vi "RW_test_fullcycle.vi"() -> ()   [LabVIEW 2018]
panel:
  in  "voltage 2":dbl
  out "error out":errorcluster caption="Error OUT"
  in  "milliseconds to wait":u32=500
  in  "Rotating Wall Parameters":T1={"Start Frequency"=25000.0, "Stop Frequency"=26000.0, "Sweep Time"=10.0, "Amplitude"=0.0, "Phase (ch.1)"=0.0, "Phase (Ch.2)"=90.0} {"Sweep Time" format="%.4f"; "Phase (Ch.2)" min=-1800.0 max=1800.0 step=0.1 format="%.3f"; "Phase (ch.1)" min=-1800.0 max=1800.0 step=0.1 format="%.3f"; "Stop Frequency" format="%#.5p"; "Start Frequency" format="%#.5p"; "Amplitude" min=0.0 max=4.0 format="%.3f"}
  in  "voltage":dbl=2.0
  in  "VISAsession":refnum<visa-resource-name>="wavefactoryU5"
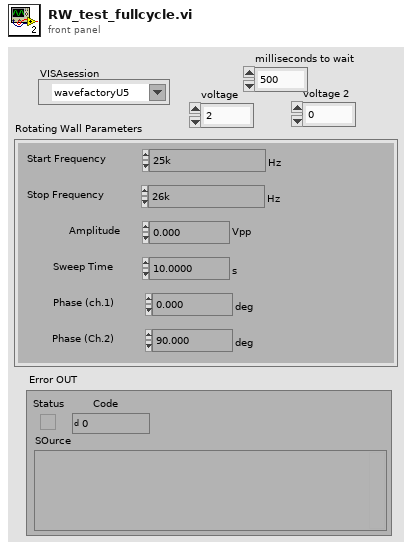
[diagram p1: front panel]
types:
  T1 = cluster{"Start Frequency":dbl, "Stop Frequency":dbl, "Sweep Time":dbl, "Amplitude":dbl, "Phase (ch.1)":dbl, "Phase (Ch.2)":dbl}
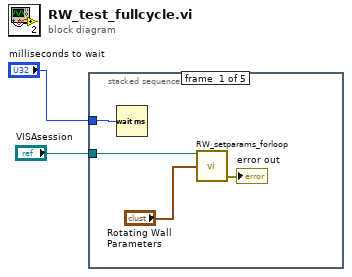
[diagram p0: block diagram]
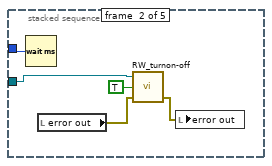
[diagram p2: hidden frame]
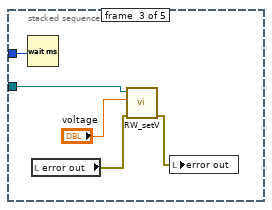
[diagram p3: hidden frame]
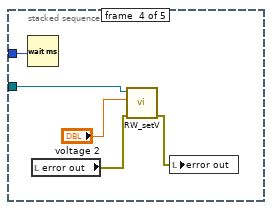
[diagram p4: hidden frame]
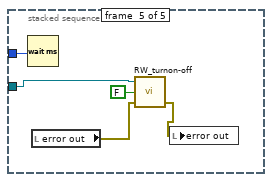
[diagram p5: hidden frame]
diagram:
  n1 = stacked-sequence {
    tunnel: "VISAsession" -> [w6 w10 w16 w21 w25]
    tunnel: "milliseconds to wait" -> [w4 w9 w15 w20 w24]
    frame #0 {
      n2 = Wait (ms)(milliseconds to wait=w4) -> ()  [unwired: 1 out]
      n3 = call "RW_setparams_forloop.vi"("Rotating Wall Parameters"="Rotating Wall Parameters", "VISAsession"=w6) -> ("error out"=→"error out":errorcluster)  [unwired: 2 in, 1 out]
    }
    frame #1 {
      n4 = Wait (ms)(milliseconds to wait=w9) -> ()  [unwired: 1 out]
      n5 = local read "error out"() -> (w8:errorcluster)
      n6 = call "RW_turnon-off.vi"("error in (no error)"=w8, "On/Off"=TRUE, "VISAsession"=w10) -> ("error out"=w7:errorcluster)  [unwired: 1 in, 1 out]
      n7 = local write "error out"(w7) -> ()
    }
    frame #2 {
      n8 = Wait (ms)(milliseconds to wait=w15) -> ()  [unwired: 1 out]
      n9 = local read "error out"() -> (w13:errorcluster)
      n10 = call "RW_setV.vi"("error in (no error)"=w13, "voltage"="voltage", "VISAsession"=w16) -> ("error out"=w12:errorcluster)  [unwired: 8 in]
      n11 = local write "error out"(w12) -> ()
    }
    frame #3 {
      n12 = Wait (ms)(milliseconds to wait=w20) -> ()  [unwired: 1 out]
      n13 = local read "error out"() -> (w18:errorcluster)
      n14 = call "RW_setV.vi"("error in (no error)"=w18, "voltage"="voltage 2", "VISAsession"=w21) -> ("error out"=w17:errorcluster)  [unwired: 8 in]
      n15 = local write "error out"(w17) -> ()
    }
    frame #4 {
      n16 = Wait (ms)(milliseconds to wait=w24) -> ()  [unwired: 1 out]
      n17 = local read "error out"() -> (w22:errorcluster)
      n18 = call "RW_turnon-off.vi"("error in (no error)"=w22, "On/Off"=FALSE, "VISAsession"=w25) -> ("error out"=w23:errorcluster)  [unwired: 1 in, 1 out]
      n19 = local write "error out"(w23) -> ()
    }
  }
